vi "getTel.vi"(8 "error in (no error)":errorcluster, 10 "telQueueServerTimeout":i32, 11 "tcpServerTel in":refnum<class "TcpServerTel.lvclass">) -> (0 "error out":errorcluster, 1 "Remaining Elements":i32, 2 "tcpPacket":string, 3 "tcpServerTel out":refnum<class "TcpServerTel.lvclass">)   [LabVIEW 2018, in "TcpServerTel.lvclass"]
doc: "Get telemetry elements one by one from queue."
uses:
  TcpServerTel.lvclass
  TcpServerTel.lvclass/TcpServerTel.ctl
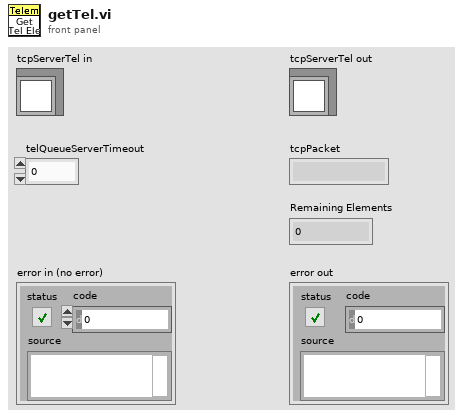
[diagram p1: front panel]
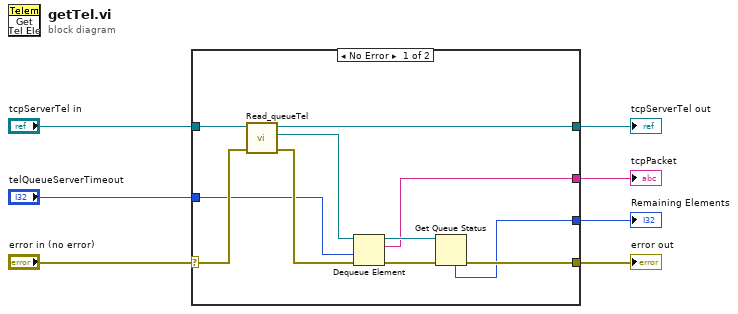
[diagram p0: block diagram]
diagram:
  n1 = case shown="No Error" "error in (no error)" {
    selector: "error in (no error)" -> [w16 w20]
    tunnel: "tcpServerTel in" -> [w18 w19]
    tunnel: [w17 w19] -> w6
    tunnel: [w10 w20] -> w4
    tunnel: "telQueueServerTimeout" -> [w11 _]
    tunnel: [w9 _] -> w2
    tunnel: [w8 _] -> w1
    frame No Error {
      n2 = call "Read_queueTel.vi"("error in (no error)"=w16, "TcpServerTel in"=w18) -> ("error out"=w13:errorcluster, "queueTel"=w12:refnum<queue>, "TcpServerTel out"=w17:refnum<class "TcpServerTel.lvclass">)  [unwired: 7 in]
      n3 = Dequeue Element(queue=w12, timeout in ms (-1)=w11, error in (no error)=w13) -> (queue out=w14:refnum<queue>, element=w8:string, error out=w15:errorcluster)  [unwired: 1 out]
      n4 = Get Queue Status(queue=w14, error in (no error)=w15) -> (error out=w10:errorcluster, # elements in queue=w9:i32)  [unwired: 1 in, 6 out]
    }
    frame Error {
    }
  }
  "error out" <- w4
  "tcpServerTel out" <- w6
  "tcpPacket" <- w1
  "Remaining Elements" <- w2
